vi "Localization.vi"(11 "未本地化":string) -> (3 "本地化":string)   [LabVIEW 2017, in "TPP demo V2启动器.lvlib"]
panel:
  in  "已本地化数组":string[](array[string])=["TPP demo V2", "正在加载应用程序...", "正在读取配置文件...", "完成！", "TPP demo\nV2", "当前操作："]
  in  "DNL_未本地化数组":string[](array[string])=["Splash Screen Title", "Loading Application", "Reading Configuration", "Done!", "App Name", "Current Action:"]
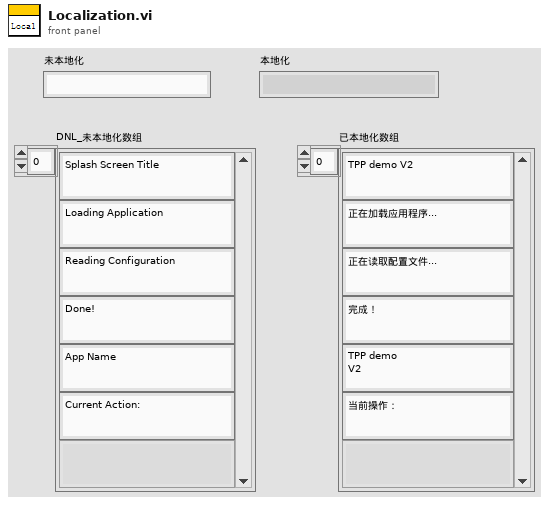
[diagram p1: front panel]
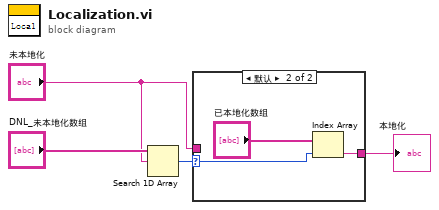
[diagram p0: block diagram]
diagram:
  n1 = Search 1D Array(1D array="DNL_未本地化数组", element="未本地化") -> (index of element=w2:i32)  [unwired: 1 in]
  n2 = case shown="默认" w2 {
    selector: w2 -> [_ w6]
    tunnel: [w5 w7] -> w3
    tunnel: "未本地化" -> [w5 _]
    frame ..-1 {
    }
    frame Default {
      n3 = Index Array(array="已本地化数组", index=w6) -> (element=w7:string)
    }
  }
  "本地化" <- w3
